vi "TSM Set TEDS Microphone DAQmx Tasks.vi"(0 "TSM context":T1, 1 "current excitation (4mA)":dbl=0.004 format="%#_6p", 5 "Sampling Rate (Hz)":dbl format="%#_6pHz", 7 "Samples per channel":i32=1000, 9 "max dB SPL":dbl=132.0 format="%.2p", 11 "error in (no error)":errorcluster, 12 "input config (differential)":i32(ring)=10106 items=["default"=-1, "RSE"=10083, "NRSE"=10078, "Differential"=10106, "Pseudodifferential"=12529]) -> (15 "error out":errorcluster)   [LabVIEW 2020]
doc: "Use this VI to initialize AI tasks for TEDS Microphones on connected NI-DAQmx instruments in the pin map associated with the test program."
uses:
  <vilib>/NI_TestStand_SemiconductorModule/NI_TestStand_Semiconductor_Module.lvlibp/PinMap/General/SemiconductorModuleContext.ctl
  <vilib>/DAQmx/create/channels.llb/DAQmx Create Channel (TEDS-AI-Sound Pressure-Microphone).vi
  <vilib>/DAQmx/configure/timing.llb/DAQmx Timing (Sample Clock).vi
  <vilib>/NI_TestStand_SemiconductorModule/NI_TestStand_Semiconductor_Module.lvlibp
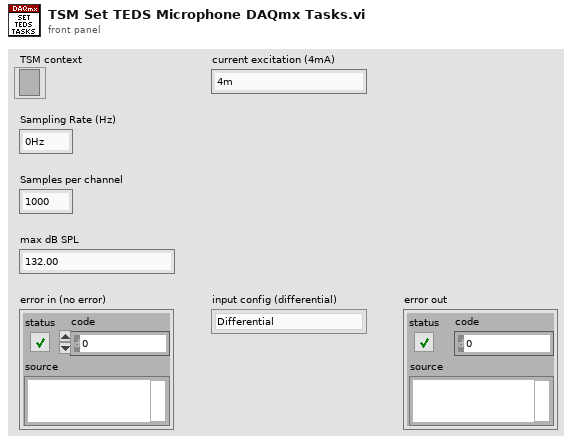
[diagram p1: front panel]
types:
  T1 = typedef "NI_TestStand_Semiconductor_Module.lvlibp/SemiconductorModuleContext.ctl" = refnum<k7>
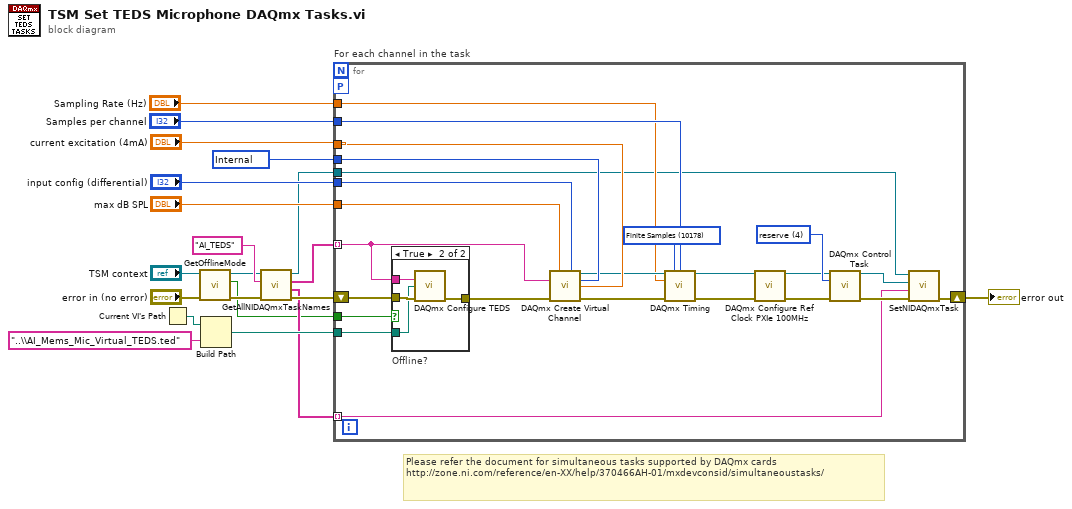
[diagram p0: block diagram]
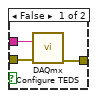
[diagram p2: hidden frame]
diagram:
  w17 = 10200 items=["Internal"=10200, "External"=10167, "None"=10230] ("current excitation source")
  # "Please refer the document for simultaneous tasks supported by DAQmx cards\nhttp://zone.ni.com/reference/en-XX/help/370466AH-01/mxdevconsid/simultaneoustasks/"
  n1 = Current VI's Path() -> (path=w12:path)
  n2 = call <vilib>:"GetOfflineMode.vi"("error in (no error)"="error in (no error)", "Semiconductor Module Context"="TSM context") -> ("error out"=w13:errorcluster, "Is Semiconductor Module In Offline Mode"=w2:bool, "Semiconductor Module Context Out"=w14:T1)  [unwired: 7 in]
  n3 = Build Path(base path=w12, name or relative path="..\\AI_Mems_Mic_Virtual_TEDS.ted") -> (appended path=w10:path)
  n4 = call <vilib>:"GetAllNIDAQmxTaskNames.vi"("error in (no error)"=w13, "Task Type"="AI_TEDS", "Semiconductor Module Context"=w14) -> ("error out"=w6:errorcluster, "Task Names"=w4:string[], "Channel Lists"=w7:string[], "Semiconductor Module Context Out"=w5:T1)  [unwired: 5 in]
  n5 = for "For each channel in the task" {
    tunnel: "max dB SPL" -> [w44]
    tunnel: w17 -> [w43]
    tunnel: "current excitation (4mA)" -> [w42]
    tunnel: "input config (differential)" -> [w41]
    shift-right: [w25] -> w3
    shift-left: w6 -> [w40]
    tunnel: w7 -> [w38] mode=indexing
    tunnel: w2 -> [w37]
    tunnel: w10 -> [w36]
    tunnel: "Samples per channel" -> [w32]
    tunnel: "Sampling Rate (Hz)" -> [w31]
    tunnel: w5 -> [w27]
    tunnel: w4 -> [w26] mode=indexing
    workers-P: _ -> [_]
    w30 = 4 items=["verify"=2, "reserve"=4, "commit"=3, "unreserve"=5, "abort"=6] ("action")
    w33 = 10178 items=["Finite Samples"=10178, "Continuous Samples"=10123, "Hardware Timed Single Point"=12522] ("sample mode")
    n6 = case "Offline?" shown="True" w37 {
      tunnel: w40 -> [w47 w51]
      tunnel: [w46 w50] -> w39
      tunnel: w38 -> [w45 w49]
      tunnel: w36 -> [_ w48]
      frame False {
        n7 = call <vilib>:"DAQmx Configure TEDS.vi"("physical channel"=w45, "error in"=w47) -> ("error out"=w46:errorcluster)  [unwired: 13 in]
      }
      frame True {
        n8 = call <vilib>:"DAQmx Configure TEDS.vi"("physical channel"=w49, "virtual TEDS file"=w48, "error in"=w51) -> ("error out"=w50:errorcluster)  [unwired: 12 in]
      }
    }
    n9 = call-poly <vilib>:"DAQmx Create Virtual Channel.vi"("maximum sound pressure level"=w44, "input terminal configuration"=w41, "physical channels"=w38, "current excitation source"=w43, "current excitation value"=w42, "error in"=w39) -> ("task out"=w34:refnum<k21>, "error out"=w35:errorcluster)  [unwired: 8 in]
    n10 = call-poly <vilib>:"DAQmx Timing.vi"("task/channels in"=w34, "sample mode"=w33, "samples per channel"=w32, "rate"=w31, "error in"=w35) -> ("task out"=w24:refnum<k21>, "error out"=w23:errorcluster)  [unwired: 9 in]
    n11 = call "DAQmx Configure Ref Clock PXIe 100MHz.vi"("DAQmx Task In"=w24, "error in (no error)"=w23) -> ("DAQmx Task Out"=w22:refnum<k21>, "error out"=w21:errorcluster)  [unwired: 12 in]
    n12 = call <vilib>:"DAQmx Control Task.vi"("task/channels in"=w22, "action"=w30, "error in"=w21) -> ("task out"=w28:refnum<k21>, "error out"=w29:errorcluster)  [unwired: 11 in]
    n13 = call <vilib>:"SetNIDAQmxTask.vi"("error in (no error)"=w29, "Task Name"=w26, "DAQmx Task"=w28, "Semiconductor Module Context"=w27) -> ("error out"=w25:errorcluster)  [unwired: 6 in, 1 out]
  }
  "error out" <- w3
